vi "Resize Panel to Pane.vi"(8 "error in (no error)":errorcluster, 11 "MediatorBusMonitor In":refnum<class "MediatorBusMonitor.lvclass">) -> (0 "error out":errorcluster, 3 "MediatorBusMonitor Out":refnum<class "MediatorBusMonitor.lvclass">)   [LabVIEW 2015, in "Mediator.lvlib" / "MediatorBusMonitor.lvclass"]
doc: "<License>\nCopyright © 2017 Composed Systems, LLC | All rights reserved\nwww.composed.io\n\nAuthor: Ethan Stern <ethan.stern@composed.io>\n\nThis software is provided \"AS IS\" WITHOUT WARRANTIES, either express or implied, AND IS FOR EDUCATIONAL PURPOSES ONLY.\n</License>"
uses:
  MediatorBusMonitor.lvclass
  MediatorBusMonitor.lvclass/MediatorBusMonitor.ctl
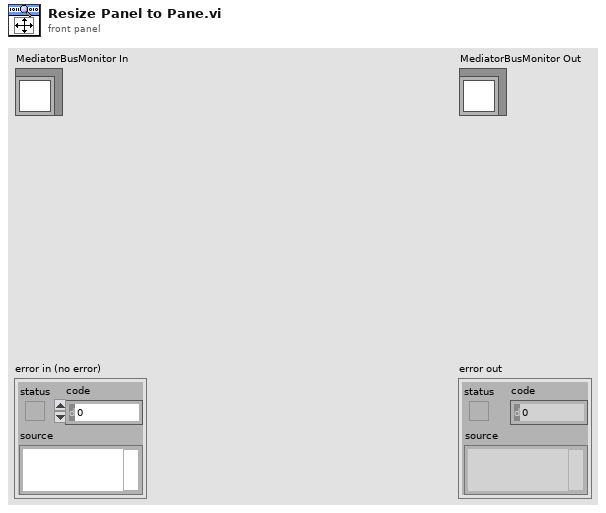
[diagram p1: front panel]
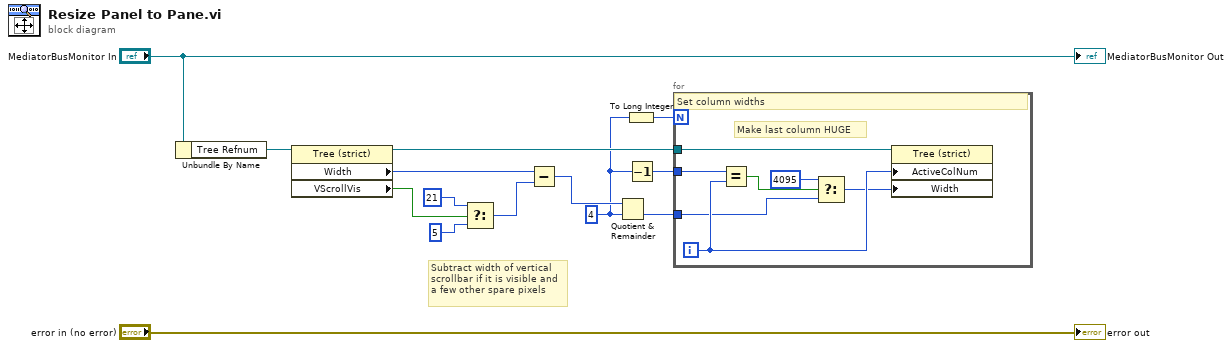
[diagram p0: block diagram]
diagram:
  w2 = u32 4 ("y")
  # "Subtract width of vertical\nscrollbar if it is visible and\na few other spare pixels"
  n1 = Unbundle By Name("MediatorBusMonitor In") -> ("Tree Refnum"=w12:refnum<vi>)
  n2 = property class="Tree (strict)"(reference=w12) -> (reference out=w10:refnum<vi>, "Width"=w9:u32, "VScrollVis"=w8:bool)  [unwired: 1 in, 1 out]
  n3 = Select(t=u32 21, s=w8, f=u32 5) -> (s? t:f=w4:u32)
  n4 = Subtract(x=w9, y=w4) -> (x-y=w5:u32)
  n5 = Quotient & Remainder(x=w5, y=w2) -> (floor(x/y)=w3:u32)  [unwired: 1 out]
  n6 = To Long Integer(number=w2) -> (32bit integer=w11:i32)
  n7 = Decrement(x=w2) -> (x-1=w1:u32)
  n8 = for {
    N: w11 -> [_]
    tunnel: w10 -> [w21]
    tunnel: w3 -> [w17]
    tunnel: w1 -> [w19]
    i -> [w20]
    # "Make last column HUGE"
    # "Set column widths"
    n9 = Equal?(x=w19, y=w20) -> (x = y?=w18:bool)
    n10 = Select(t=u32 4095, s=w18, f=w17) -> (s? t:f=w16:u32)
    n11 = property class="Tree (strict)"(reference=w21, "ActiveColNum"=w20, "Width"=w16) -> ()  [unwired: 1 in, 2 out]
  }
  "error out" <- "error in (no error)"
  "MediatorBusMonitor Out" <- "MediatorBusMonitor In"
